vi "determine rtdsc freq.vi"() -> ()   [LabVIEW 2024]
uses:
  8ebdbc22-dfbb-47a3-99c3-91fb7999871a.vi
  Neuer Ordner (2)/PerfCountersExperiment/RtdscLV.dll
panel:
  out "Current Rdtsc Value":u64=6573235728850
  out "increments in one second":u64=3600656847
  # "0,278"
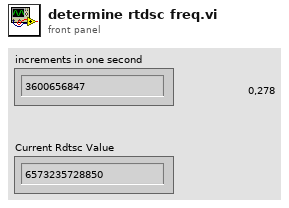
[diagram p1: front panel]
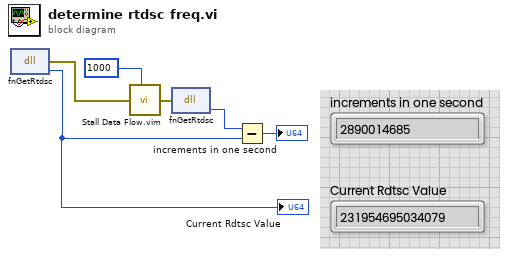
[diagram p0: block diagram]
diagram:
  n1 = dll-call lib="C:/Users/Andrey/Desktop/Neuer Ordner (2)/PerfCountersExperiment/RtdscLV.dll" fn="fnGetRtdsc"() -> (error out=w6:errorcluster, "return type"=w1:u64)  [unwired: 3 in, 1 out]
  "Current Rdtsc Value" <- w1
  n2 = call "Stall Data Flow.vim"("value in"=w6, "milliseconds to wait"=u32 1000) -> ("value out"=w4:errorcluster)  [unwired: 1 out]
  n3 = dll-call lib="C:/Users/Andrey/Desktop/Neuer Ordner (2)/PerfCountersExperiment/RtdscLV.dll" fn="fnGetRtdsc"(error in=w4) -> ("return type"=w3:u64)  [unwired: 2 in, 2 out]
  n4 = Subtract(x=w3, y=w1) -> (x-y=→"increments in one second":u64)
